vi "Write BRAND SELECTED TI.vi"(8 "error in (no error)":errorcluster, 10 "BRAND SELECTED":enum16{"NXP", "TI", "SIMULATED"}(ring), 11 "TI in":refnum<class "TI.lvclass">) -> (0 "error out":errorcluster, 3 "TI out":refnum<class "TI.lvclass">)   [LabVIEW 2019, in "TI.lvclass"]
uses:
  TI.lvclass
  TI.lvclass/TI.ctl
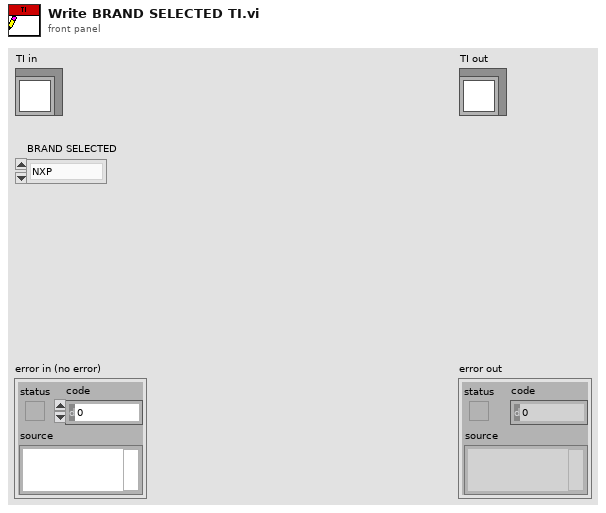
[diagram p1: front panel]
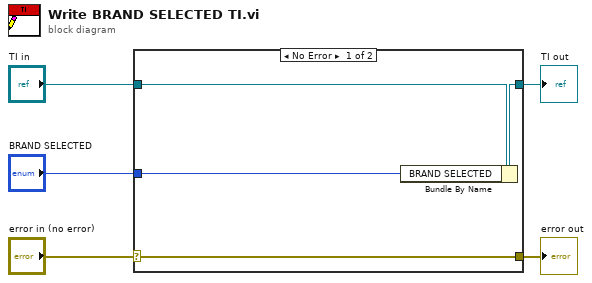
[diagram p0: block diagram]
diagram:
  n1 = case shown="No Error" "error in (no error)" {
    selector: "error in (no error)" -> [w9 w10]
    tunnel: [w9 w10] -> w4
    tunnel: [w7 w11] -> w2
    tunnel: "TI in" -> [w8 w11]
    tunnel: "BRAND SELECTED" -> [w6 _]
    frame No Error {
      n2 = Bundle By Name(cluster=w8, "BRAND SELECTED"=w6) -> (w7:refnum<class "TI.lvclass">)
    }
    frame Error {
    }
  }
  "error out" <- w4
  "TI out" <- w2
